vi "Apply DMA Configuration.vi"(7 "DMA Settings":T1 {"DMA Host Buffer" items=["1 Second"=1, "2 Seconds"=2, "5 Seconds"=5, "10 Seconds"=10]; "dt" format="%#_p"; "Update Rate" items=["1 Hz"=1, "2 Hz"=2, "5 Hz"=5, "10 Hz"=10]}, 8 "error in (no error)":errorcluster, 11 "Item Ref in":T4 format="%.0x") -> (0 "error out":errorcluster)   [LabVIEW 2019, in "FPGA Addon System Explorer.lvlib"]
uses:
  FPGA Addon System Explorer.lvlib
  <vilib>/NI VeriStand/Custom Device API/Custom Device Item Ref.ctl
  Addon Shared/Types/DMA Settings.ctl
  Addon Shared/Types/Delacing Scheme.ctl
  Addon Shared/Types/DMA Acquisition Mode.ctl
  Addon Shared/Types/FG Action.ctl
  Addon Shared/SubVIs/Constants.vi
  <vilib>/NI VeriStand/Custom Device API/NI VeriStand - Get Item Property.vi
  <vilib>/NI VeriStand/Custom Device API/Get Item Property (U32).vi
  <vilib>/NI VeriStand/Custom Device API/Get Item Property (Double).vi
  <vilib>/NI VeriStand/Custom Device API/NI VeriStand - Set Item Property.vi
  <vilib>/NI VeriStand/Custom Device API/Set Item Property (U32).vi
  <vilib>/NI VeriStand/Custom Device API/Set Item Property (Double).vi
  Addon Shared/FPGA Addon Shared.lvlib
  <vilib>/NI VeriStand/Custom Device API/Custom Device API.lvlib
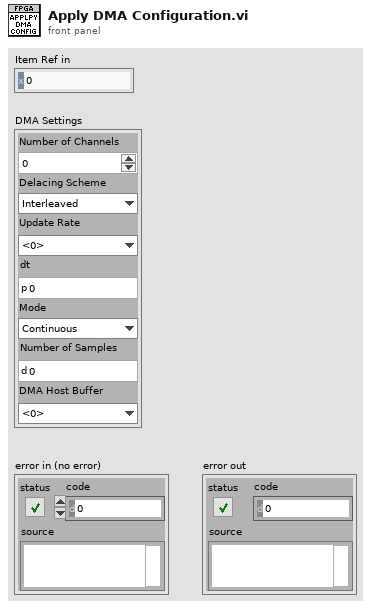
[diagram p1: front panel]
types:
  T1 = typedef "FPGA Addon Shared.lvlib/DMA Settings.ctl" = cluster{"Number of Channels":u8, "Delacing Scheme":T2, "Update Rate":u32, "dt":dbl, "Mode":T3, "Number of Samples":u32, "DMA Host Buffer":u32}
  T2 = typedef "FPGA Addon Shared.lvlib/Delacing Scheme.ctl" = enum8{"Interleaved", "Bitpacked"}
  T3 = typedef "FPGA Addon Shared.lvlib/DMA Acquisition Mode.ctl" = enum8{"Continuous", "Triggered Finite"}
  T4 = typedef "Custom Device API.lvlib/Custom Device Item Ref.ctl" = u64
  T5 = typedef "FPGA Addon Shared.lvlib/FG Action.ctl" = enum8{"GET", "SET"}
  T6 = typedef "Custom Device API.lvlib/Custom Device Item Info.ctl" = cluster{"Name":string, "Is Channel":bool, "GUID":string, "Is Waveform":bool}
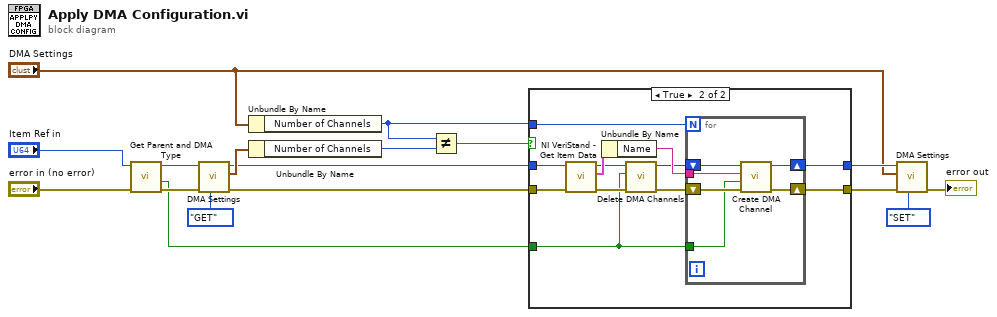
[diagram p0: block diagram]
diagram:
  n1 = call "Get Parent and DMA Type.vi"("error in (no error)"="error in (no error)", "Node Ptr"="Item Ref in") -> ("error out"=w3:errorcluster, "Input?"=w1:bool, "Item Ref out"=w2:T4)  [unwired: 6 in, 1 out]
  n2 = call "DMA Settings.vi"("Action"=FG_Action."GET", "error in (no error)"=w3, "Item Ref"=w2) -> ("error out"=w12:errorcluster, "DMA Settings"=w17:T1, "Item Ref out"=w13:T4)  [unwired: 6 in]
  n3 = Unbundle By Name("DMA Settings") -> ("Number of Channels"=w6:u8)
  n4 = Unbundle By Name(w17) -> ("Number of Channels"=w14:u8)
  n5 = Not Equal?(x=w6, y=w14) -> (x != y?=w16:bool)
  n6 = case shown="True" w16 {
    tunnel: w1 -> [_ w20]
    tunnel: [w18 w29] -> w10
    tunnel: w12 -> [w18 w25]
    tunnel: w13 -> [w19 w26]
    tunnel: w6 -> [_ w28]
    tunnel: [w19 w27] -> w15
    frame False {
    }
    frame True {
      n7 = call <vilib>:"NI VeriStand - Get Item Data.vi"("error in (no error)"=w25, "Item Ref in"=w26) -> ("error out"=w24:errorcluster, "Item Info"=w31:T6, "Item Ref out"=w23:T4)  [unwired: 7 out]
      n8 = Unbundle By Name(w31) -> ("Name"=w30:string)
      n9 = call "Delete DMA Channels.vi"("error in (no error)"=w24, "Input?"=w20, "Item Ref in"=w23) -> ("error out"=w21:errorcluster, "Section Ref out"=w22:T4)  [unwired: 7 in]
      n10 = for {
        N: w28 -> [_]
        tunnel: w30 -> [w34]
        shift-right: [w37] -> w29
        shift-left: w21 -> [w36]
        shift-right: [w33] -> w27
        shift-left: w22 -> [w35]
        tunnel: w20 -> [w32]
        n11 = call "Create DMA Channel.vi"("error in (no error)"=w36, "Input?"=w32, "Name"=w34, "Section Ref in"=w35) -> ("error out"=w37:errorcluster, "Parent Ref out"=w33:T4)  [unwired: 6 in]
      }
    }
  }
  n12 = call "DMA Settings.vi"("Action"=FG_Action."SET", "error in (no error)"=w10, "DMA Settings"="DMA Settings", "Item Ref"=w15) -> ("error out"=→"error out":errorcluster)  [unwired: 5 in, 2 out]
